vi "Convert Image to U8 and send to FPGA.vi"(6 "FPGA VI Reference Out 2":refnum<k20>, 7 "Maximum Pixels per Write":i32=480000, 8 "FPGA VI Reference Out 2":refnum<k20>, 9 "Range":cluster{"Lower Value":u8, "Upper Value":u8}, 10 "Image Dst":T1, 11 "ImageIn":T1) -> (0 "error out":errorcluster, 1 "Timimngs":u32[](array[numeric]), 3 "Image Out":T1)   [LabVIEW 2015]
uses:
  <vilib>/vision/Image Controls.llb/IMAQ Image.ctl
  <vilib>/Utility/error.llb/Error Cluster From Error Code.vi
  <vilib>/rvi/errors/niLvFpgaAdjustHostInterfaceError.vi
  <vilib>/rvi/interface/nirviReadWriteControl/nirviReadWriteControl.xnode
  <vilib>/rvi/interface/nirviMethod/nirviMethod.xnode
  <vilib>/vision/NI_Vision_Development_Module.lvlib
  <vilib>/visionFPGA/NI_VDM_FPGA_Basics.lvlib
  <vilib>/visionFPGA/Basics/Image Transfer to Target/IMAQ FPGA Image Transfer to Target U8.vi
  NiFpgaLv.dll
  <vilib>/rvi/interface/Simulation/niFpgaSimulationCallBeginRW.vi
  <vilib>/FPGAPlugInAG/Dynamic/niLvFpga_WriteFifo_Dynamic.vi
  <vilib>/rvi/errors/niLvFpgaMergeErrorWithErrorCode.vi
panel:
  in  "Color Plane":i32(ring) items=["Red", "Green", "Blue", "Hue", "Saturation", "Luminance", "Value", "Intensity"]
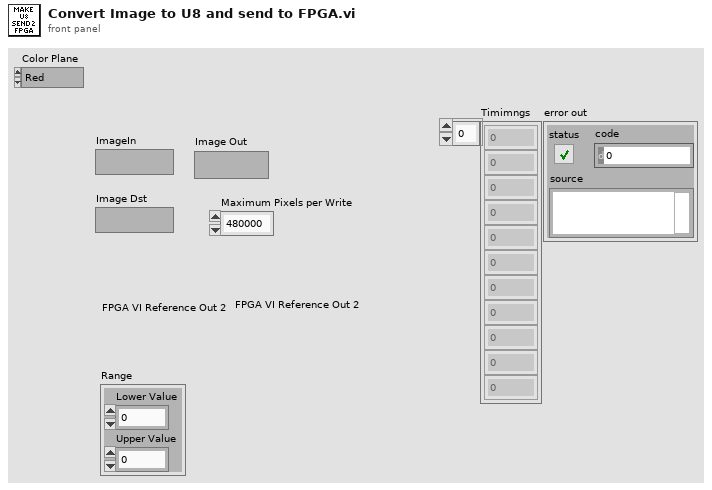
[diagram p1: front panel]
types:
  T1 = typedef "IMAQ Image.ctl" = refnum<image>
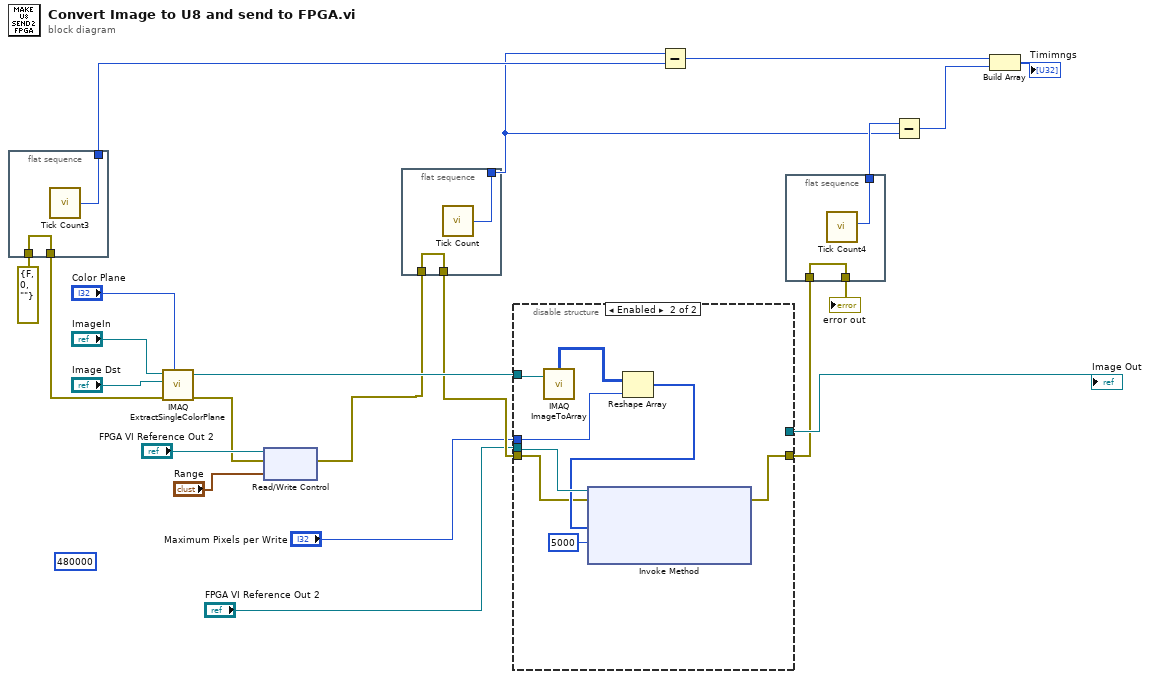
[diagram p0: block diagram]
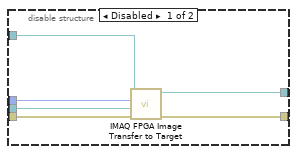
[diagram p2: hidden frame]
diagram:
  (unwired) 480000 ("Maximum Pixels per Write")
  n1 = flat-sequence {
    tunnel: errorcluster {"status"=FALSE, "code"=0, "source"=""} ("error out") -> [w24]
    tunnel: [w24] -> w19
    tunnel: [w23] -> w17
    frame #0 {
      n2 = call "Tick Count3"() -> ("Tick Count(mSec)"=w23:u32)
    }
  }
  n3 = call "IMAQ ExtractSingleColorPlane"("Color Plane"="Color Plane", "error in (no error)"=w19, "Image Dst"="Image Dst", "Image Src"="ImageIn") -> ("error out"=w5:errorcluster, "Image Dst Out"=w9:T1)  [unwired: 6 out]
  n4 = xnode "Read/Write Control"("FPGA VI Reference In"="FPGA VI Reference Out 2", "error in"=w5, "Range"="Range") -> ("error out"=w4:errorcluster)  [unwired: 1 out]
  n5 = flat-sequence {
    tunnel: w4 -> [w26]
    tunnel: [w26] -> w6
    tunnel: [w25] -> w12
    frame #0 {
      n6 = call "Tick Count"() -> ("Tick Count(mSec)"=w25:u32)
    }
  }
  n7 = disable-structure shown="Enabled" {
    disable-tunnel: w9 -> [w32 w40]
    disable-tunnel: [w31 _] -> w8
    disable-tunnel: [w30 w33] -> w7
    disable-tunnel: w6 -> [w29 w34]
    disable-tunnel: "Maximum Pixels per Write" -> [w28 w38]
    disable-tunnel: "FPGA VI Reference Out 2" -> [w27 w37]
    frame Disabled {
      n8 = call-poly <vilib>:"IMAQ FPGA Image Transfer to Target.vi"("error in (no error)"=w29, "DMA FIFO Reference In"=w27, "Maximum Pixels per Write"=w28, "Image"=w32) -> ("error out"=w30:errorcluster, "Image Out"=w31:T1)  [unwired: 5 in, 1 out]
    }
    frame Enabled {
      n9 = call "IMAQ ImageToArray"("Image"=w40) -> ("Image Pixels (U8)"=w39:u8[][])  [unwired: 3 in, 4 out]
      n10 = Reshape Array(w39, w38) -> (w36:u8[])
      n11 = xnode "Invoke Method"("FPGA VI Reference In"=w37, "error in"=w34, "Data"=w36, "Timeout (ms)"=5000) -> ("error out"=w33:errorcluster)  [unwired: 2 out]
    }
  }
  "Image Out" <- w8
  n12 = Subtract(x=w12, y=w17) -> (x-y=w16:u32)
  n13 = flat-sequence {
    tunnel: [w42] -> w14
    tunnel: w7 -> [w41]
    tunnel: [w41] -> w1
    frame #0 {
      n14 = call "Tick Count4"() -> ("Tick Count(mSec)"=w42:u32)
    }
  }
  n15 = Subtract(x=w14, y=w12) -> (x-y=w13:u32)
  n16 = Build Array(w16, w13) -> (→"Timimngs":u32[])
  "error out" <- w1
